vi "exponente.vi"() -> ()   [LabVIEW 2013]
panel:
  out "Portencia":dbl
  out "Exponente":dbl
  out "Base":dbl
  # "Generar la base y el exponente con numeros de 1-10\nluego generar la potencia usando el ciclo for."
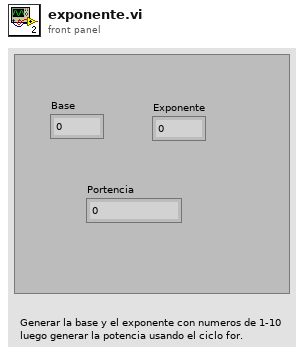
[diagram p1: front panel]
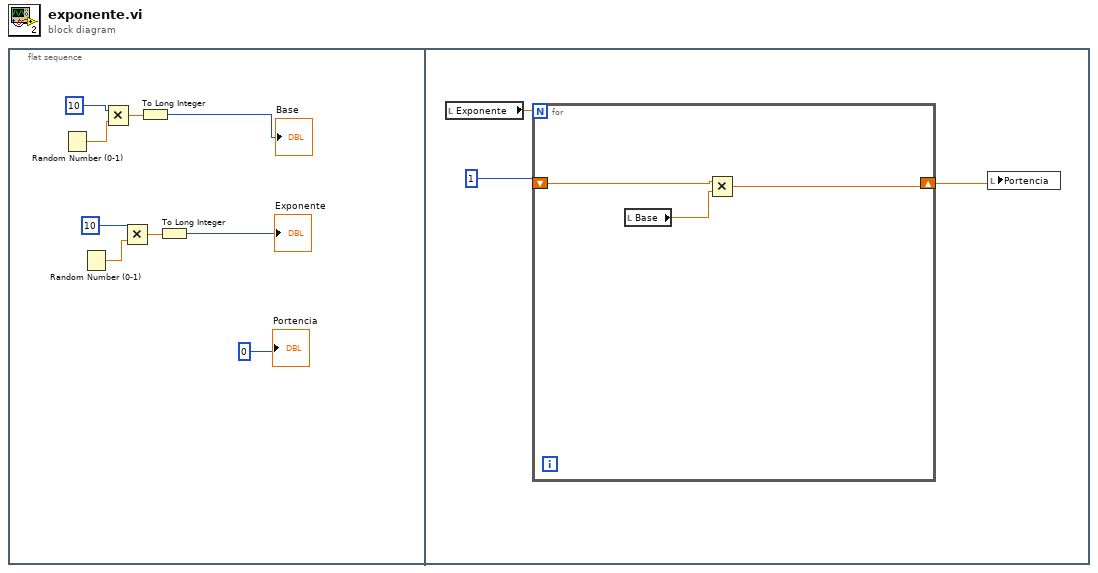
[diagram p0: block diagram]
diagram:
  n1 = flat-sequence {
    frame #0 {
      n2 = Random Number (0-1)() -> (number: 0 to 1=w7:dbl)
      n3 = Random Number (0-1)() -> (number: 0 to 1=w4:dbl)
      n4 = Multiply(x=10, y=w7) -> (x*y=w9:dbl)
      n5 = Multiply(x=10, y=w4) -> (x*y=w3:dbl)
      n6 = To Long Integer(number=w9) -> (32bit integer=→"Base":i32)
      n7 = To Long Integer(number=w3) -> (32bit integer=→"Exponente":i32)
      "Portencia" <- 0
    }
    frame #1 {
      n8 = local read "Exponente"() -> (w12:dbl)
      n9 = for {
        N: w12 -> [_]
        shift-right: [w13] -> w10
        shift-left: 1 -> [w15]
        n10 = local read "Base"() -> (w14:dbl)
        n11 = Multiply(x=w15, y=w14) -> (x*y=w13:dbl)
      }
      n12 = local write "Portencia"(w10) -> ()
    }
  }
